vi "Set Top Level.vi"(8 "error in":errorcluster, 10 "Project Reference":refnum<vi>, 11 "VI Reference":refnum<vi>) -> (0 "error out":errorcluster)   [LabVIEW 2020]
doc: "Mark a VI in the project as the top level VI TopVI."
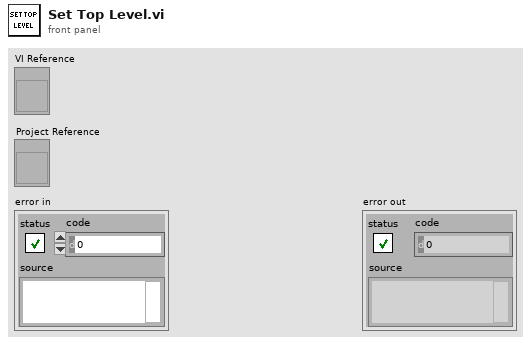
[diagram p1: front panel]
types:
  T1 = enum32{"invalid VI type", "Standard VI", "Control VI", "Global VI", "Polymorphic VI", "Configuration VI", "SubSystem", "Facade VI", "Method VI", "Statechart Diagram VI"}
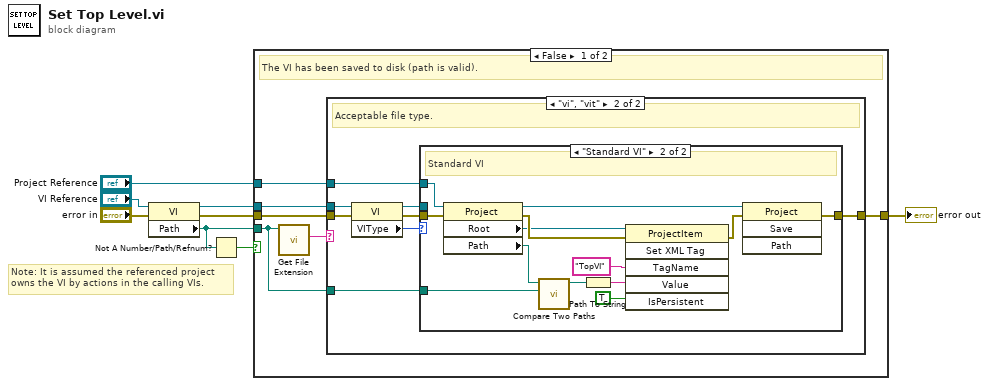
[diagram p0: block diagram]
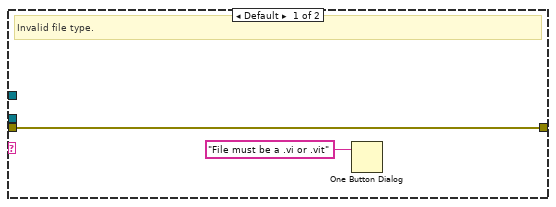
[diagram p2: hidden frame]
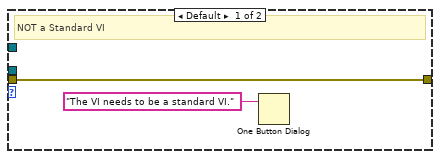
[diagram p3: hidden frame]
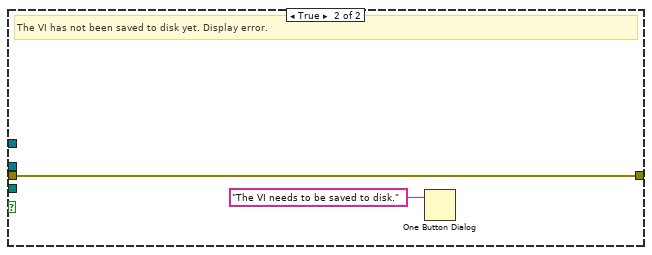
[diagram p4: hidden frame]
diagram:
  # "Note: It is assumed the referenced project owns the VI by actions in the calling VIs."
  n1 = property class="VI"(reference="VI Reference", error in="error in") -> (reference out=w1:refnum<vi>, error out=w6:errorcluster, "Path"=w4:path)
  n2 = Not A Number/Path/Refnum?(number/path/refnum=w4) -> (NaN/Path/Refnum?=w5:bool)
  n3 = case shown="False" w5 {
    tunnel: w6 -> [w14 w41]
    tunnel: [w13 w41] -> w8
    tunnel: w4 -> [w11 _]
    tunnel: "Project Reference" -> [w12 _]
    tunnel: w1 -> [w9 _]
    frame False {
      # "The VI has been saved to disk (path is valid)."
      n4 = call <vilib>:"Get File Extension.vi"("file"=w11) -> ("lowercase file extension"=w10:string)  [unwired: 6 in, 4 out]
      n5 = case shown="\"vi\", \"vit\"" w10 {
        tunnel: w14 -> [w16 w23]
        tunnel: [w16 w24] -> w13
        tunnel: w12 -> [_ w21]
        tunnel: w11 -> [_ w20]
        tunnel: w9 -> [_ w19]
        frame Default {
          # "Invalid file type."
          n6 = One Button Dialog(message="File must be a .vi or .vit") -> ()  [unwired: 1 in, 1 out]
        }
        frame "vi", "vit" {
          # "Acceptable file type."
          n7 = property class="VI"(reference=w19, error in=w23) -> (reference out=w17:refnum<vi>, error out=w22:errorcluster, "VIType"=w18:T1)
          n8 = case shown="\"Standard VI\"" w18 {
            tunnel: w22 -> [w26 w38]
            tunnel: [w26 w39] -> w24
            tunnel: w21 -> [_ w34]
            tunnel: w20 -> [_ w35]
            tunnel: w17 -> [_ _]
            frame Default {
              # "NOT a Standard VI"
              n9 = One Button Dialog(message="The VI needs to be a standard VI.") -> ()  [unwired: 1 in, 1 out]
            }
            frame "Standard VI" {
              # "Standard VI"
              n10 = property class="Project"(reference=w34, error in=w38) -> (reference out=w30:refnum<vi>, error out=w37:errorcluster, "Root"=w33:refnum<vi>, "Path"=w29:path)
              n11 = call <vilib>:"Compare Two Paths.vi"("Path 2"=w35, "Path 1"=w29) -> ("Relative Path from 1 to 2"=w28:path)  [unwired: 6 in, 3 out]
              n12 = Path To String(path=w28) -> (string=w27:string)
              n13 = invoke class="ProjectItem" method="Set XML Tag"(reference=w33, error in=w37, "TagName"="TopVI" ("Tag Name"), "Value"=w27, "IsPersistent"=TRUE ("Is Persistent")) -> (error out=w36:errorcluster)  [unwired: 1 in, 5 out]
              n14 = invoke class="Project" method="Save"(reference=w30, error in=w36) -> (error out=w39:errorcluster)  [unwired: 2 in, 3 out]
            }
          }
        }
      }
    }
    frame True {
      # "The VI has not been saved to disk yet. Display error."
      n15 = One Button Dialog(message="The VI needs to be saved to disk.") -> ()  [unwired: 1 in, 1 out]
    }
  }
  "error out" <- w8
